vi "Parse Navigation Results.vi"(11 "String":string) -> ()   [LabVIEW 2017, in "VisionHW.lvlib"]
uses:
  VisionHW.lvlib
  <vilib>/regexp/Match Regular Expression.xnode
panel:
  out "submatch 8":string
  in  "Regex":string="(Object:\\s+w=\\s+(\\d+\\.\\d+)\\s+h=\\s+(\\d+\\.\\d+)\\s+r=\\s+(\\d+\\.\\d+)\\s+x=\\s+([-]*\\d+)\\s+y=\\s+([-]*\\d+)\\s+d=\\s+(\\d+)\\s+){0,1}RN:\\s+([-]{0,1}\\d+)"
  out "submatch 7":string
  out "submatch 6":string
  out "submatch 5":string
  out "submatch 4":string
  out "submatch 3":string
  out "submatch 2":string
  out "submatch 1":string
  # "Object: w= 1.2 h= 3.4 r= 5.6 x= -7 y= -8 d= 9    RN: -100"
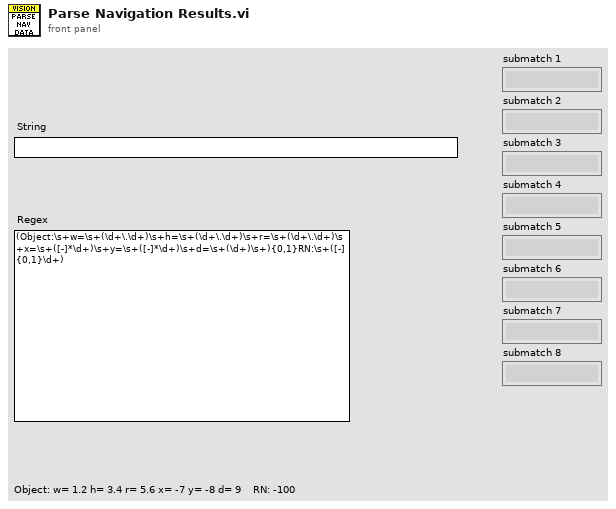
[diagram p1: front panel]
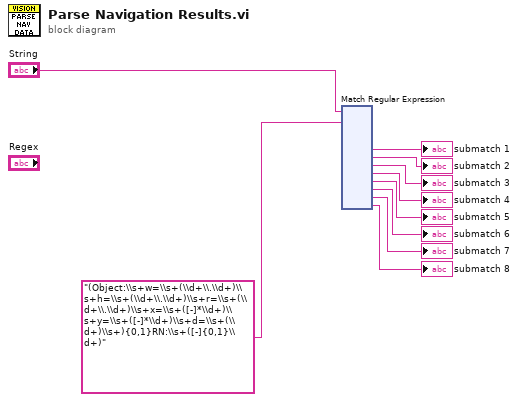
[diagram p0: block diagram]
diagram:
  n1 = xnode "Match Regular Expression"("input string"="String", "regular expression"="(Object:\\s+w=\\s+(\\d+\\.\\d+)\\s+h=\\s+(\\d+\\.\\d+)\\s+r=\\s+(\\d+\\.\\d+)\\s+x=\\s+([-]*\\d+)\\s+y=\\s+([-]*\\d+)\\s+d=\\s+(\\d+)\\s+){0,1}RN:\\s+([-]{0,1}\\d+)") -> ("submatch 1"=→"submatch 1":string, "submatch 2"=→"submatch 2":string, "submatch 3"=→"submatch 3":string, "submatch 4"=→"submatch 4":string, "submatch 5"=→"submatch 5":string, "submatch 6"=→"submatch 6":string, "submatch 7"=→"submatch 7":string, "submatch 8"=→"submatch 8":string)  [unwired: 4 in, 5 out]
